vi "AcqHydData.vi"(6 "Time Out (ms)":dbl=1000.0 min=-1.0, 7 "Scope":bool, 10 "Handle Cluster 2":T1, 11 "Handle Cluster 1":T1) -> (3 "Data in Volts":sgl[][][](array[numeric]))   [LabVIEW 2022 SP3]
uses:
  ScanningControl/Digitizers/GaGe/-GageUtils/GageGlobals.vi
  <instrlib>/LeCroy Wave Series/LeCroy Wave Series.lvlib
panel:
  out "Percent Complete":u8(slide) scale=0.0..100.0
  out "Status":string
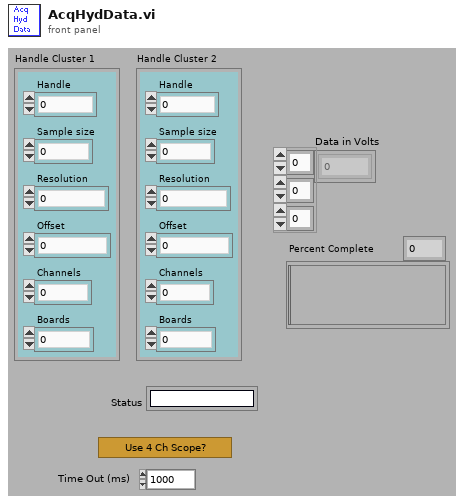
[diagram p1: front panel]
types:
  T1 = cluster{"Handle":u32, "Sample size":u32, "Resolution":i32, "Offset":i32, "Channels":u32, "Boards":u32}
  T2 = cluster{"Sample Rate":dbl, "Clock Mode":enum16{"Internal", "External", "Reference"}, "Mode":string, "Depth":dbl, "Segment Size":dbl, "Trigger Timeout":dbl, "Trigger Holdoff":dbl, "Trigger Delay":dbl}
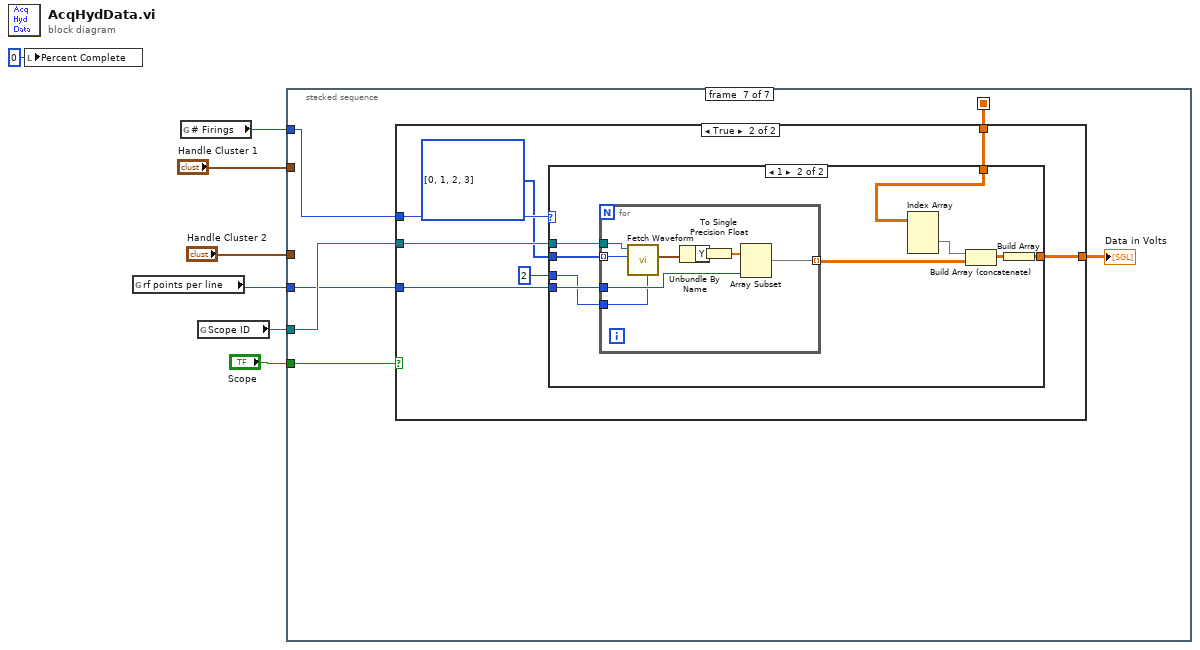
[diagram p0: block diagram]
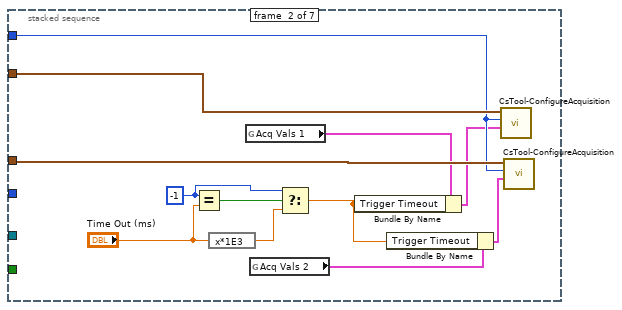
[diagram p3: hidden frame]
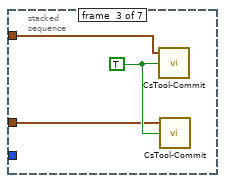
[diagram p4: hidden frame]
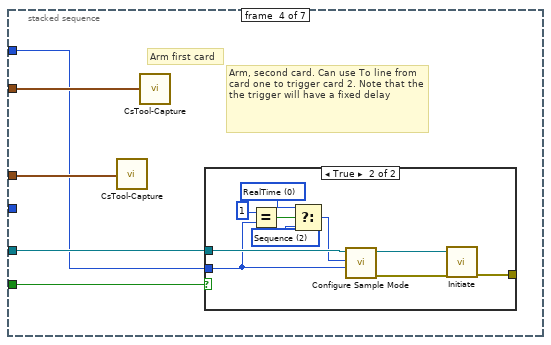
[diagram p5: hidden frame]
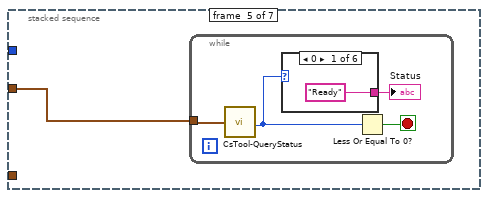
[diagram p7: hidden frame]
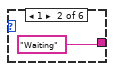
[diagram p8: hidden frame]
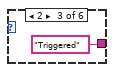
[diagram p9: hidden frame]
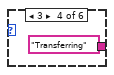
[diagram p10: hidden frame]
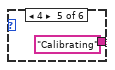
[diagram p11: hidden frame]
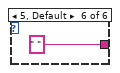
[diagram p12: hidden frame]
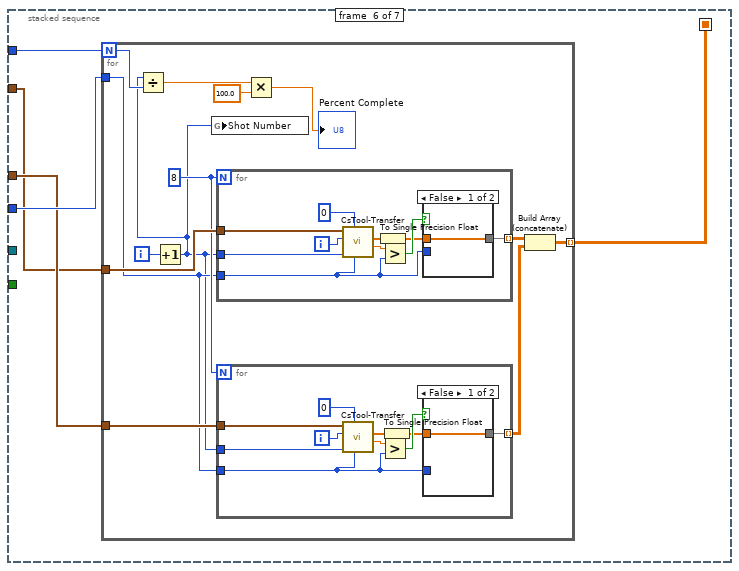
[diagram p13: hidden frame]
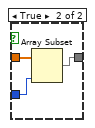
[diagram p14: hidden frame]
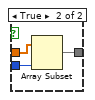
[diagram p15: hidden frame]
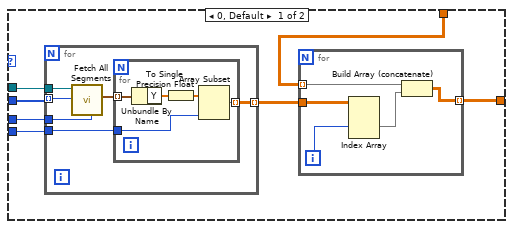
[diagram p17: hidden frame]
diagram:
  n1 = local write "Percent Complete"(u8 0 ("Percent Complete")) -> ()
  n2 = global read "GageGlobals.vi" "rf points per line"() -> (w4:i32)
  n3 = global read "GageGlobals.vi" "# Firings"() -> (w6:u16)
  n4 = global read "GageGlobals.vi" "Scope ID"() -> (w3:refnum<visa-resource-name>)
  n5 = stacked-sequence {
    seq-local: [_ _ _ _ _ w49 _] -> [_ _ _ _ _ _ w96]
    tunnel: "Handle Cluster 1" -> [_ w19 w22 w27 w38 w50 _]
    tunnel: w6 -> [_ w17 _ w23 _ w53 w99]
    tunnel: w4 -> [_ _ _ _ _ w52 w97]
    tunnel: "Handle Cluster 2" -> [_ w18 w20 w26 _ w51 _]
    tunnel: w3 -> [_ _ _ w25 _ _ w98]
    tunnel: "Scope" -> [_ _ _ w24 _ _ w100]
    frame #0 {
    }
    frame #1 {
      w8 = -1
      n6 = Equal?(x=w8, y="Time Out (ms)") -> (x = y?=w12:bool)
      n7 = expression code="x*1E3"("Time Out (ms)") -> (w11:dbl)
      n8 = global read "GageGlobals.vi" "Acq Vals 1"() -> (w16:T2)
      n9 = global read "GageGlobals.vi" "Acq Vals 2"() -> (w14:T2)
      n10 = Select(t=w8, s=w12, f=w11) -> (s? t:f=w10:dbl)
      n11 = Bundle By Name(cluster=w16, "Trigger Timeout"=w10) -> (w15:T2)
      n12 = Bundle By Name(cluster=w14, "Trigger Timeout"=w10) -> (w13:T2)
      n13 = call <userlib>:"CsTool-ConfigureAcquisition.vi"("Handle Cluster"=w19, "Segment Count (1)"=w17, "Acquisition"=w15) -> ()  [unwired: 2 in, 1 out]
      n14 = call <userlib>:"CsTool-ConfigureAcquisition.vi"("Handle Cluster"=w18, "Segment Count (1)"=w17, "Acquisition"=w13) -> ()  [unwired: 2 in, 1 out]
    }
    frame #2 {
      w21 = TRUE ("Coerce Flag (f)")
      n15 = call <userlib>:"CsTool-Commit.vi"("Coerce Flag (f)"=w21, "Handle Cluster"=w22) -> ()  [unwired: 1 in, 2 out]
      n16 = call <userlib>:"CsTool-Commit.vi"("Coerce Flag (f)"=w21, "Handle Cluster"=w20) -> ()  [unwired: 1 in, 2 out]
    }
    frame #3 {
      # "Arm, second card. Can use To line from card one to trigger card 2. Note that the the trigger will have a fixed delay"
      # "Arm first card"
      n17 = call <userlib>:"CsTool-Capture.vi"("Handle Cluster"=w26) -> ()  [unwired: 1 out]
      n18 = call <userlib>:"CsTool-Capture.vi"("Handle Cluster"=w27) -> ()  [unwired: 1 out]
      n19 = case shown="True" w24 {
        tunnel: w25 -> [_ w36]
        tunnel: [_ w37] -> _
        tunnel: w23 -> [_ w33]
        frame False {
        }
        frame True {
          w29 = u16 0 items=["RealTime", "RIS", "Sequence", "Roll", "WaveStream"] ("Sample Mode (0: RealTime)")
          w30 = u16 2 items=["RealTime", "RIS", "Sequence", "Roll", "WaveStream"] ("Sample Mode (0: RealTime)")
          n20 = Equal?(x=1, y=w33) -> (x = y?=w31:bool)
          n21 = Select(t=w29, s=w31, f=w30) -> (s? t:f=w28:u16)
          n22 = call <instrlib>:"Configure Sample Mode.vi"("Number of Segments (2)"=w33, "Sample Mode (0: RealTime)"=w28, "VISA resource name"=w36) -> ("error out"=w34:errorcluster, "VISA resource name out"=w35:refnum<visa-resource-name>)  [unwired: 1 in, 6 out]
          n23 = call <instrlib>:"Initiate.vi"("error in (no error)"=w34, "VISA resource name"=w35) -> ("error out"=w37:errorcluster)  [unwired: 1 in, 8 out]
        }
      }
    }
    frame #4 {
      n24 = while {
        tunnel: w38 -> [w40]
        stop <- w39 stop-if-true
        n25 = call <userlib>:"CsTool-QueryStatus.vi"("Handle Cluster"=w40) -> ("Status"=w41:i32)
        n26 = case shown="0" w41 {
          tunnel: ["Ready" "Waiting" "Triggered" "Transferring" "Calibrating" " "] -> w42
          frame 0 {
          }
          frame 1 {
          }
          frame 2 {
          }
          frame 3 {
          }
          frame 4 {
          }
          frame 5, Default {
          }
        }
        "Status" <- w42
        n27 = Less Or Equal To 0?(x=w41) -> (x <= 0?=w39:bool)
      }
    }
    frame #5 {
      n28 = for {
        N: w53 -> [w58]
        tunnel: [w61] -> w49 mode=indexing
        tunnel: w50 -> [w66]
        tunnel: w52 -> [w59]
        tunnel: w51 -> [w64]
        i -> [w65]
        w60 = 8
        n29 = Increment(x=w65) -> (x+1=w55:i32)
        n30 = Divide(x=w55, y=w58) -> (x/y=w57:dbl)
        n31 = global write "GageGlobals.vi" "Shot Number"(w55) -> ()
        n32 = for {
          N: w60 -> [_]
          tunnel: [w88] -> w63 mode=indexing
          tunnel: w66 -> [w87]
          tunnel: w59 -> [w84]
          tunnel: w55 -> [w82]
          i -> [w83]
          n33 = call <userlib>:"CsTool-Transfer.vi"("Length (4096)"=w84, "Start (0)"=0, "Segment (1)"=w82, "Channel (0)"=w83, "Handle Cluster"=w87) -> ("Actual Length"=w86:dbl, "Data in Volts"=w89:dbl[])  [unwired: 1 in, 2 out]
          n34 = To Single Precision Float(number=w89) -> (single precision float=w81:sgl[])
          n35 = Greater?(x=w86, y=w84) -> (0:w90:bool)
          n36 = case shown="False" w90 {
            tunnel: w81 -> [w91 w94]
            tunnel: [w91 w92] -> w88
            tunnel: w84 -> [_ w93]
            frame False {
            }
            frame True {
              n37 = Array Subset(array=w94, length=w93) -> (w92:sgl[])  [unwired: 1 in]
            }
          }
        }
        n38 = for {
          N: w60 -> [_]
          tunnel: [w74] -> w62 mode=indexing
          tunnel: w64 -> [w73]
          tunnel: w55 -> [w69]
          tunnel: w59 -> [w68]
          i -> [w70]
          n39 = call <userlib>:"CsTool-Transfer.vi"("Length (4096)"=w68, "Start (0)"=0, "Segment (1)"=w69, "Channel (0)"=w70, "Handle Cluster"=w73) -> ("Actual Length"=w72:dbl, "Data in Volts"=w75:dbl[])  [unwired: 1 in, 2 out]
          n40 = Greater?(x=w72, y=w68) -> (0:w76:bool)
          n41 = To Single Precision Float(number=w75) -> (single precision float=w67:sgl[])
          n42 = case shown="False" w76 {
            tunnel: w67 -> [w77 w80]
            tunnel: [w77 w78] -> w74
            tunnel: w68 -> [_ w79]
            frame False {
            }
            frame True {
              n43 = Array Subset(array=w80, length=w79) -> (w78:sgl[])  [unwired: 1 in]
            }
          }
        }
        n44 = Multiply(x=w57, y=100.0) -> (x*y=→"Percent Complete":dbl)
        n45 = Build Array (concatenate)(w63, w62) -> (w61:sgl[][])
      }
    }
    frame #6 {
      n46 = case shown="True" w100 {
        tunnel: w99 -> [_ w108]
        tunnel: w98 -> [_ w107]
        tunnel: w97 -> [_ w105]
        tunnel: w96 -> [w101 w103]
        tunnel: [w101 w102] -> w95
        frame False {
        }
        frame True {
          w106 = u16[] [0, 1, 2, 3] items=["Channel 1", "Channel 2", "Channel 3", "Channel 4", "Memory 1", "Memory 2", "Memory 3", "Memory 4", "Function 1", "Function 2", "Function 3", "Function 4", "Function 5", "Function 6", "Function 7", "Function 8", "Other"] ("Channels")
          n47 = case shown="1" w108 {
            tunnel: w107 -> [w113 w137]
            tunnel: w106 -> [w114 w140]
            tunnel: w105 -> [w115 w139]
            tunnel: 2 ("Sparsing (0: Every point)") -> [w112 w138]
            tunnel: w103 -> [w111 w136]
            tunnel: [w109 w133] -> w102
            frame 0, Default {
              n48 = for {
                tunnel: w114 -> [w124] mode=indexing
                tunnel: w115 -> [w126]
                tunnel: [w125] -> w110 mode=indexing
                tunnel: w113 -> [w123]
                tunnel: w112 -> [w121]
                n49 = call <instrlib>:"Fetch All Segments.vi"("Sparsing (0: Every point)"=w121, "Source (0: Channel 1)"=w124, "VISA resource name"=w123) -> ("Array"=w122:waveform(dbl)[])  [unwired: 4 in, 4 out]
                n50 = for {
                  tunnel: w126 -> [w130]
                  tunnel: [w129] -> w125 mode=indexing
                  tunnel: w122 -> [w128] mode=indexing
                  n51 = Unbundle By Name(w128) -> ("Y"=w131:dbl[])
                  n52 = To Single Precision Float(number=w131) -> (single precision float=w127:sgl[])
                  n53 = Array Subset(array=w127, length=w130) -> (w129:sgl[])  [unwired: 1 in]
                }
              }
              n54 = for {
                tunnel: w111 -> [w118] mode=indexing
                tunnel: w110 -> [w120]
                tunnel: [w116] -> w109 mode=indexing
                i -> [w119]
                n55 = Index Array(array=w120, index (dim 1)=w119) -> (element=w117:sgl[][])  [unwired: 2 in]
                n56 = Build Array (concatenate)(w118, w117) -> (w116:sgl[][])
              }
            }
            frame 1 {
              n57 = for {
                tunnel: w140 -> [w148] mode=indexing
                tunnel: w139 -> [w145]
                tunnel: [w144] -> w134 mode=indexing
                tunnel: w138 -> [w143]
                tunnel: w137 -> [w142]
                n58 = call <instrlib>:"Fetch Waveform.vi"("Sparsing (0: Every point)"=w143, "Source (0: Channel 1)"=w148, "VISA resource name"=w142) -> ("Waveform Graph"=w147:waveform(dbl))  [unwired: 6 in, 2 out]
                n59 = Unbundle By Name(w147) -> ("Y"=w146:dbl[])
                n60 = To Single Precision Float(number=w146) -> (single precision float=w141:sgl[])
                n61 = Array Subset(array=w141, length=w145) -> (w144:sgl[])  [unwired: 1 in]
              }
              n62 = Index Array(array=w136) -> (element=w135:sgl[][])  [unwired: 3 in]
              n63 = Build Array (concatenate)(w135, w134) -> (w132:sgl[][])
              n64 = Build Array(w132) -> (w133:sgl[][][])
            }
          }
        }
      }
      "Data in Volts" <- w95
    }
  }
